vi "GetRelayState.vi"(8 "error in (no error)":errorcluster, 10 "index":u32, 11 "device":u32) -> (0 "error out":errorcluster, 2 "function return":u32(ring), 3 "state":u32(ring) items=["IRB_RELAY_STATE_OFF", "IRB_RELAY_STATE_ON"])   [LabVIEW 2015, in "IRB.lvlib"]
doc: "irb_result IRB_EXPORT irb_get_relay_state(irb_device* device, size_t index, irb_relay_state* state);"
uses:
  IRB.lvlib
  IRB.dll
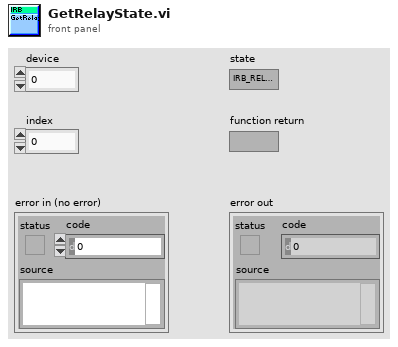
[diagram p1: front panel]
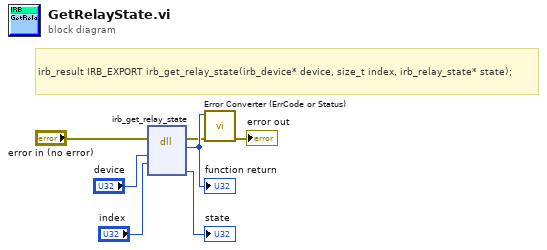
[diagram p0: block diagram]
diagram:
  # "irb_result IRB_EXPORT irb_get_relay_state(irb_device* device, size_t index, irb_relay_state* state);"
  n1 = dll-call lib="C:/LabView/IRB/x86_32/IRB.*" fn="irb_get_relay_state"(error in="error in (no error)", "device"="device", "index"="index") -> (error out=w2:errorcluster, w7:u32, "state"=→"state":u32)  [unwired: 5 in, 1 out]
  "function return" <- w7
  n2 = call "Error Converter (ErrCode or Status).vi"("error in (no error)"=w2, "error code"=w7) -> ("error out"=→"error out":errorcluster)  [unwired: 9 in]
